vi "CreateEndoHeader.vi"(8 "error in (no error)":errorcluster) -> (0 "error out":errorcluster, 3 "header":string)   [LabVIEW 2014]
uses:
  Classes/CAREX_Classes/Endoscope/WristPos.ctl
  Classes/CAREX_Classes/ForceField/TypeDef/FF_Gains.ctl
  Classes/MotorControl/TypeDef/MotorMode.ctl
  Classes/DataLogger/Data Logger.lvclass
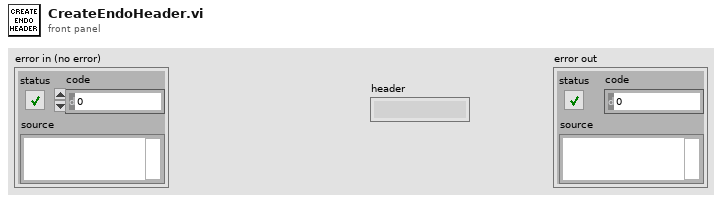
[diagram p1: front panel]
types:
  T1 = typedef "Endoscope.lvclass/WristPos.ctl" = cluster{"DistToJoint":dbl, "DownFromStick":dbl, "RightToStick":dbl}
  T2 = typedef "ForceField.lvclass/FF_Gains.ctl" = cluster{"Kn":dbl, "Dn":dbl, "Kt":dbl, "Dt":dbl, "Kd":dbl, "Ns":dbl}
  T3 = typedef "MotorControl.lvclass/MotorMode.ctl" = enum16{"Idle", "FF", "PID"}
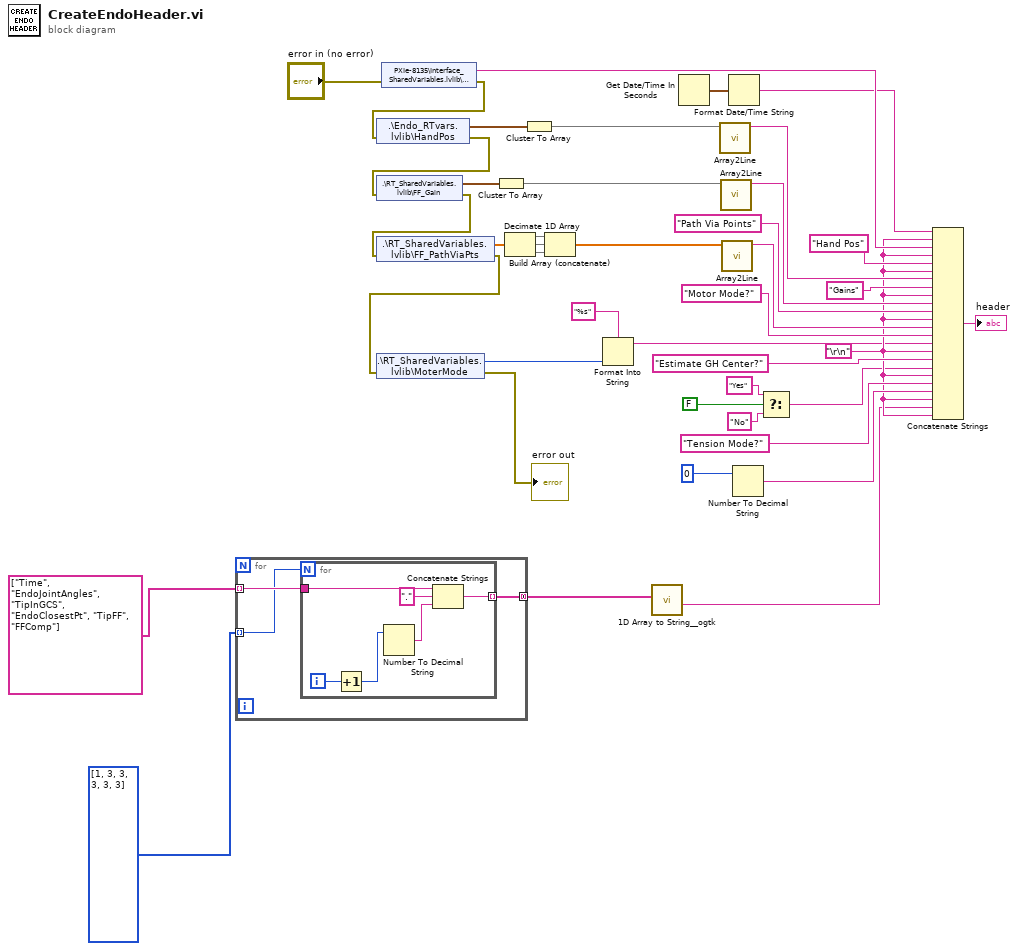
[diagram p0: block diagram]
diagram:
  w28 = "\r\n"
  n1 = for {
    tunnel: i32[] [1, 3, 3, 3, 3, 3] -> [w44] mode=indexing
    tunnel: string[] ["Time", "EndoJointAngles", "TipInGCS", "EndoClosestPt", "TipFF", "FFComp"] -> [w45] mode=indexing
    tunnel: [w43] -> w10 mode=concatenating
    n2 = for {
      N: w44 -> [_]
      tunnel: w45 -> [w51]
      tunnel: [w46] -> w43 mode=indexing
      i -> [w48]
      n3 = Increment(x=w48) -> (x+1=w47:i32)
      n4 = Number To Decimal String(number=w47) -> (decimal integer string=w49:string)  [unwired: 1 in]
      n5 = Concatenate Strings(w51, ".", w49) -> (w46:string)
    }
  }
  n6 = shared-variable "PXIe-8135\\Interface_SharedVariables.lvlib\\FileName"(error in="error in (no error)") -> (w36:string, error out=w8:errorcluster)
  n7 = shared-variable ".\\Endo_RTvars.lvlib\\HandPos"(error in=w8) -> (w19:T1, error out=w17:errorcluster)
  n8 = shared-variable ".\\RT_SharedVariables.lvlib\\FF_Gain"(error in=w17) -> (w21:T2, error out=w16:errorcluster)
  n9 = shared-variable ".\\RT_SharedVariables.lvlib\\FF_PathViaPts"(error in=w16) -> (w5:dbl[], error out=w15:errorcluster)
  n10 = shared-variable ".\\RT_SharedVariables.lvlib\\MoterMode"(error in=w15) -> (w22:T3, error out=→"error out":errorcluster)
  n11 = Cluster To Array(cluster=w21) -> (array=w20:dbl[])
  n12 = Decimate 1D Array(w5) -> (w4:dbl[], w3:dbl[], w2:dbl[])
  n13 = Cluster To Array(cluster=w19) -> (array=w18:dbl[])
  n14 = Build Array (concatenate)(w4, w3, w2) -> (w1:dbl[])
  n15 = Format Into String(format string="%s", w22) -> (resulting string=w27:string)  [unwired: 2 in, 1 out]
  n16 = call <userlib>:"1D Array to String__ogtk.vi"("Array of Strings"=w10) -> ("delimited string"=w9:string)  [unwired: 10 in]
  n17 = Get Date/Time In Seconds() -> (seconds since 1Jan1904=w34:timestamp)
  n18 = call "Array2Line.vi"("Data"=w18) -> ("String"=w29:string)  [unwired: 10 in]
  n19 = call "Array2Line.vi"("Data"=w20) -> ("String"=w38:string)  [unwired: 10 in]
  n20 = call "Array2Line.vi"("Data"=w1) -> ("String"=w40:string)  [unwired: 10 in]
  n21 = Format Date/Time String(seconds (now)=w34) -> (date/time string=w35:string)  [unwired: 2 in]
  n22 = Number To Decimal String(number=0) -> (decimal integer string=w31:string)  [unwired: 1 in]
  n23 = Select(t="Yes" ("format string"), s=FALSE, f="No" ("format string")) -> (s? t:f=w23:string)
  n24 = Concatenate Strings(w35, w28, w36, w28, "Hand Pos" ("string"), w28, w29, "Gains" ("string"), w28, w38, "Path Via Points" ("string"), w28, w40, "Motor Mode?" ("string"), w27, w28, "Estimate GH Center?" ("string"), w23, w28, "Tension Mode?" ("string"), w31, w28, w9, w28) -> (→"header":string)
